vi "Support_MergeErrors.vi"(2 "error in 1":errorcluster, 3 "error in 2":errorcluster, 4 "error in 3":errorcluster, 5 "Error array":errorcluster[](array[cluster])) -> (16 "error out":errorcluster, 17 "All error out":errorcluster[](array[cluster]))   [LabVIEW 2020]
doc: "Searches for errors in the incoming errorclusters. First error1 then error2 and 3, last errorarray."
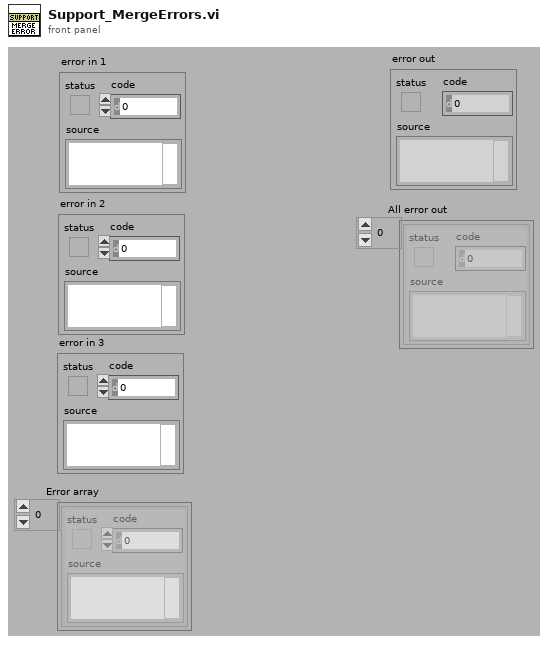
[diagram p1: front panel]
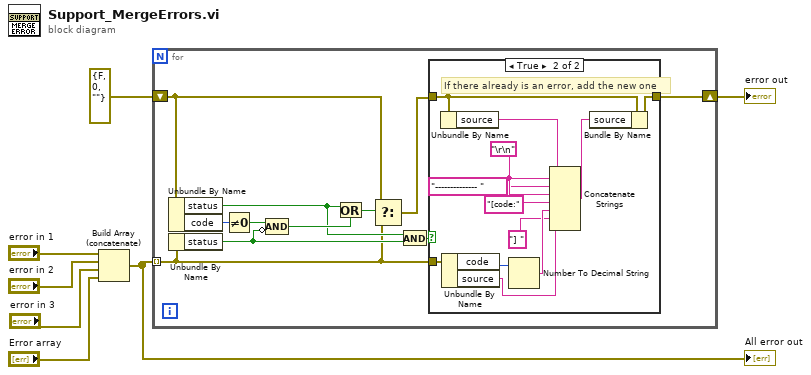
[diagram p0: block diagram]
diagram:
  n1 = Build Array (concatenate)("error in 1", "error in 2", "error in 3", "Error array") -> (w3:errorcluster[])
  "All error out" <- w3
  n2 = for {
    tunnel: w3 -> [w8] mode=indexing
    shift-right: [w12] -> w4
    shift-left: errorcluster {"status"=FALSE, "code"=0, "source"=""} ("error in (no error)") -> [w18]
    n3 = Unbundle By Name(w18) -> ("status"=w10:bool, "code"=w16:i32)
    n4 = Unbundle By Name(w8) -> ("status"=w11:bool)
    n5 = Not Equal To 0?(x=w16) -> (x != 0?=w15:bool)
    n6 = Compound Arithmetic op=AND(w15, invert w11) -> (w14:bool)
    n7 = Or(x=w10, y=w14) -> (x .or. y?=w17:bool)
    n8 = Select(t=w18, s=w17, f=w8) -> (s? t:f=w13:errorcluster)
    n9 = And(x=w10, y=w11) -> (x .and. y?=w9:bool)
    n10 = case shown="True" w9 {
      tunnel: w13 -> [w19 w30]
      tunnel: [w19 w31] -> w12
      tunnel: w8 -> [_ w29]
      frame False {
      }
      frame True {
        w21 = "\r\n"
        # "If there already is an error, add the new one"
        n11 = Unbundle By Name(w30) -> ("source"=w22:string)
        n12 = Unbundle By Name(w29) -> ("code"=w27:i32, "source"=w23:string)
        n13 = Number To Decimal String(number=w27) -> (decimal integer string=w25:string)  [unwired: 1 in]
        n14 = Concatenate Strings(w22, w21, "-------------- ", w21, "[code:" ("Substring"), w25, "] " ("Substring"), w23) -> (w28:string)
        n15 = Bundle By Name(cluster=w30, "source"=w28) -> (w31:errorcluster)
      }
    }
  }
  "error out" <- w4
